vi "FindMax.vi"() -> ()   [LabVIEW 2020]
panel:
  out "element":string
  out "max value":i32
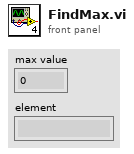
[diagram p1: front panel]
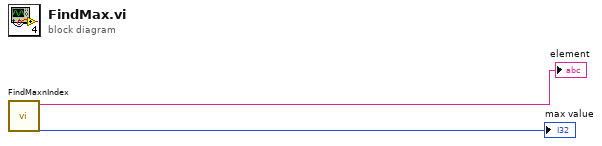
[diagram p0: block diagram]
diagram:
  n1 = call "FindMaxnIndex.vi"() -> ("Numeric"=→"max value":i32, "String"=→"element":string)  [unwired: 10 in]
